vi "Build.vi"(9 "XYZTheta":dbl[](array[numeric]), 10 "Pattern Coordinates":dbl[][](array[numeric]), 11 "CAD Dispense in":refnum<class "CAD Dispense.lvclass">) -> (1 "Starting Coordinates":dbl[](array[numeric]), 3 "CAD Dispense out":refnum<class "CAD Dispense.lvclass">)   [LabVIEW 2020, in "CAD Dispense.lvclass"]
uses:
  CAD Dispense.lvclass
  CAD Dispense.lvclass/CAD Dispense.ctl
  <vilib>/Analysis/coordinate.llb/2D Cartesian Coordinate Rotation (Scalar).vi
  <vilib>/Analysis/NI_AALPro.lvlib
panel:
  out "array w/ subset deleted 2":T1(array[cluster])
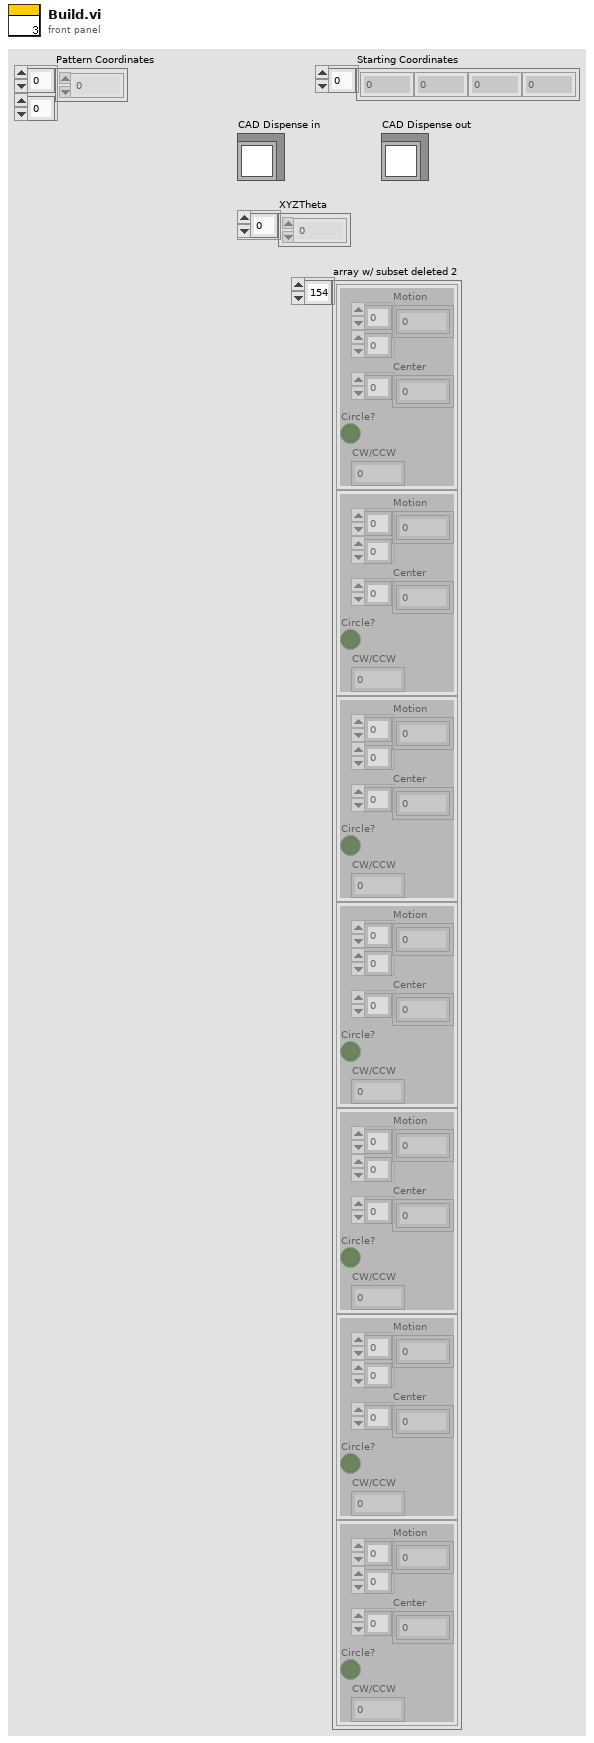
[diagram p1: front panel]
types:
  T1 = cluster{"Motion":dbl[][], "Center":dbl[], "Circle?":bool, "CW/CCW":dbl}[]
  T2 = cluster{"Motion":dbl[][], "Center":dbl[], "Circle?":bool, "CW/CCW":dbl}
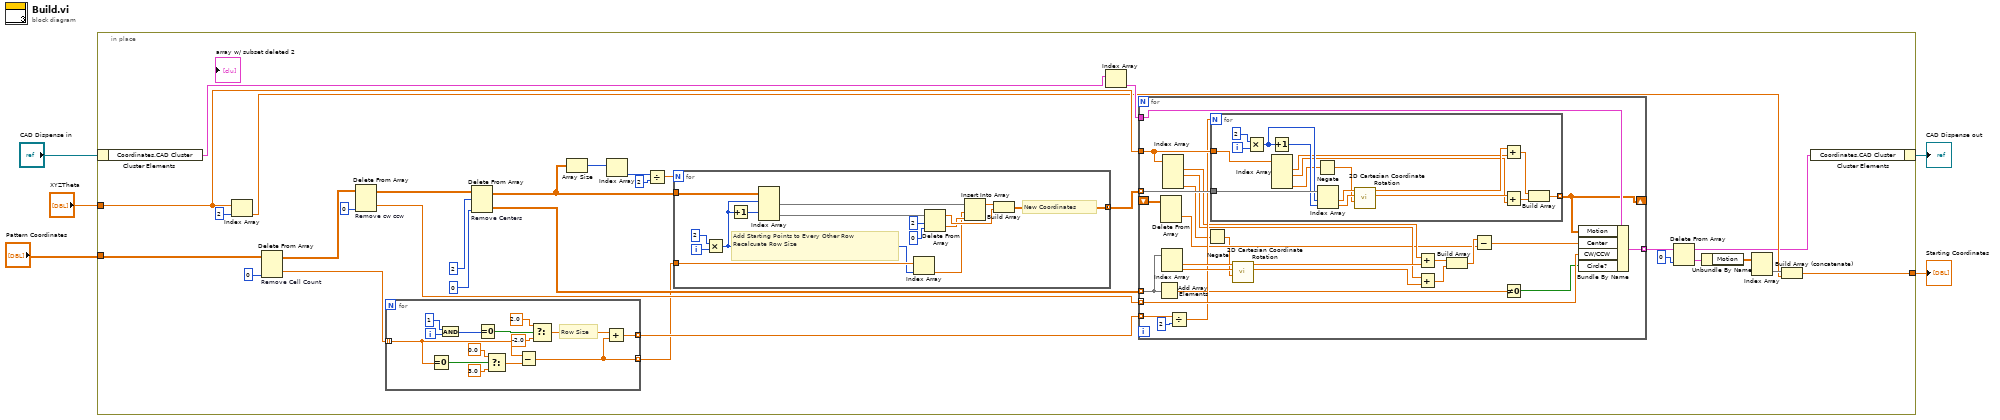
[diagram p0: block diagram]
diagram:
  n1 = in-place {
    in-place-border: "XYZTheta" -> [w10]
    in-place-border: "Pattern Coordinates" -> [w22]
    in-place-border: [w7] -> w3
    n2 = in-place-cluster #1("CAD Dispense in") -> ("Coordinates.CAD Cluster"=w24:T1)
    n3 = Index Array(array=w10, index=2) -> (element=w8:dbl)
    n4 = Delete From Array "Remove Cell Count"(array=w22, index (col)=0 ("disabled index (col)")) -> (deleted portion=w18:dbl[], array with subset deleted=w29:dbl[][])  [unwired: 2 in]
    n5 = Delete From Array "Remove cw ccw"(array=w29, index (col)=0 ("disabled index (col)")) -> (deleted portion=w34:dbl[], array with subset deleted=w30:dbl[][])  [unwired: 2 in]
    n6 = for {
      tunnel: w18 -> [w45] mode=indexing
      tunnel: [w37] -> w17 mode=indexing
      tunnel: [w36] -> w16 mode=indexing
      i -> [w38]
      # "Row Size"
      n7 = Equal To 0?(x=w45) -> (x = 0?=w46:bool)
      n8 = And(x=1, y=w38) -> (x .and. y?=w41:i32)
      n9 = Equal To 0?(x=w41) -> (x = 0?=w39:bool)
      n10 = Select(t=0.0, s=w46, f=3.0) -> (s? t:f=w49:dbl)
      n11 = Subtract(x=w45, y=w49) -> (x-y=w36:dbl)
      n12 = Select(t=2.0, s=w39, f=-2.0) -> (s? t:f=w42:dbl)
      n13 = Add(x=w42, y=w36) -> (x+y=w37:dbl)
    }
    n14 = Delete From Array "Remove Centers"(array=w30, length=2, index (col)=0 ("disabled index (col)")) -> (deleted portion=w35:dbl[][], array with subset deleted=w31:dbl[][])  [unwired: 1 in]
    n15 = Array Size(array=w31) -> (size(s)=w32:i32[])
    n16 = Index Array(array=w32) -> (element=w21:i32)  [unwired: 1 in]
    n17 = Divide(x=w21, y=2) -> (x/y=w19:dbl)
    n18 = for {
      N: w19 -> [_]
      tunnel: w31 -> [w107]
      tunnel: [w99] -> w33 mode=concatenating
      tunnel: w16 -> [w94]
      i -> [w100]
      # "New Coordinates"
      # "Add Starting Points to Every Other Row\nRecalcuate Row Size"
      n19 = Multiply(x=2, y=w100) -> (x*y=w93:i32)
      n20 = Increment(x=w93) -> (x+1=w95:i32)
      n21 = Index Array(array=w107, index (row) #1=w93, index (row) #2=w95) -> (element #1=w103:dbl[], element #2=w105:dbl[])  [unwired: 2 in]
      n22 = Index Array(array=w94, index=w93) -> (element=w96:dbl)
      n23 = Delete From Array(array=w105, length=2, index=0) -> (deleted portion=w97:dbl[], array with subset deleted=w101:dbl[])
      n24 = Insert Into Array(array=w103, index=w96, new element=w97) -> (w102:dbl[])
      n25 = Build Array(w102, w101) -> (w99:dbl[][])
    }
    n26 = Index Array(array=w24) -> (element=w23:T2)  [unwired: 1 in]
    n27 = for {
      tunnel: w17 -> [w73] mode=indexing
      tunnel: w33 -> [w68] mode=indexing
      tunnel: w34 -> [w71] mode=indexing
      tunnel: w35 -> [w67] mode=indexing
      tunnel: w10 -> [w74]
      tunnel: w23 -> [w72]
      tunnel: [w69] -> w13 mode=indexing
      shift-right: [w50] -> _
      shift-left: _ -> [w56]
      n28 = Add Array Elements(numeric array=w67) -> (sum=w53:dbl)
      n29 = Delete From Array(array=w56) -> (deleted portion=w55:dbl[])  [unwired: 3 in, 1 out]
      n30 = Index Array(array=w67) -> (element #1=w66:dbl, element #2=w65:dbl)  [unwired: 2 in]
      n31 = Index Array(array=w74) -> (element #1=w63:dbl, element #2=w58:dbl, element #4=w52:dbl)  [unwired: 4 in, 1 out]
      n32 = Divide(x=w73, y=2) -> (x/y=w64:dbl)
      n33 = Negate(x=w52) -> (-x=w51:dbl)
      n34 = for {
        N: w64 -> [_]
        tunnel: w68 -> [w92]
        tunnel: [w78] -> w50 mode=indexing
        tunnel: w74 -> [w88]
        i -> [w79]
        n35 = Multiply(x=2, y=w79) -> (x*y=w90:i32)
        n36 = Increment(x=w90) -> (x+1=w89:i32)
        n37 = Index Array(array=w88) -> (element #1=w81:dbl, element #2=w80:dbl, element #4=w77:dbl)  [unwired: 4 in, 1 out]
        n38 = Negate(x=w77) -> (-x=w76:dbl)
        n39 = Index Array(array=w92, index #1=w90, index #2=w89) -> (element #1=w84:dbl, element #2=w83:dbl)
        n40 = call-poly <vilib>:"2D Cartesian Coordinate Rotation.vi"("theta"=w76, "y"=w83, "x"=w84) -> ("y out"=w87:dbl, "x out"=w82:dbl)  [unwired: 6 in, 1 out]
        n41 = Add(x=w82, y=w81) -> (x+y=w86:dbl)
        n42 = Add(x=w87, y=w80) -> (x+y=w85:dbl)
        n43 = Build Array(w86, w85) -> (w78:dbl[])
      }
      n44 = call-poly <vilib>:"2D Cartesian Coordinate Rotation.vi"("theta"=w51, "y"=w65, "x"=w66) -> ("y out"=w60:dbl, "x out"=w62:dbl)  [unwired: 6 in, 1 out]
      n45 = Add(x=w63, y=w62) -> (x+y=w61:dbl)
      n46 = Add(x=w58, y=w60) -> (x+y=w59:dbl)
      n47 = Build Array(w61, w59) -> (w57:dbl[])
      n48 = Subtract(x=w57, y=w55) -> (x-y=w54:dbl[])
      n49 = Not Equal To 0?(x=w53) -> (x != 0?=w70:bool)
      n50 = Bundle By Name(cluster=w72, "Motion"=w50, "Center"=w54, "CW/CCW"=w71, "Circle?"=w70) -> (w69:T2)
    }
    n51 = Delete From Array "Delete From Array"(array=w13, index=0) -> (deleted portion=w15:T2, array with subset deleted=w6:T1)  [unwired: 1 in]
    n52 = Unbundle By Name(w15) -> ("Motion"=w12:dbl[][])
    n53 = Index Array(array=w12) -> (element=w11:dbl[])  [unwired: 2 in]
    n54 = Build Array (concatenate)(w11, w8) -> (w7:dbl[])
    n55 = in-place-cluster #1("Coordinates.CAD Cluster"=w6) -> (→"CAD Dispense out":refnum<class "CAD Dispense.lvclass">)
  }
  "Starting Coordinates" <- w3
